vi "Enable-disable control.vi"(8 "error in":errorcluster, 10 "Status":T1(array[ring]), 11 "Ref array":refnum<vi>[](array[refnum])) -> (0 "error out":errorcluster)   [LabVIEW 2018]
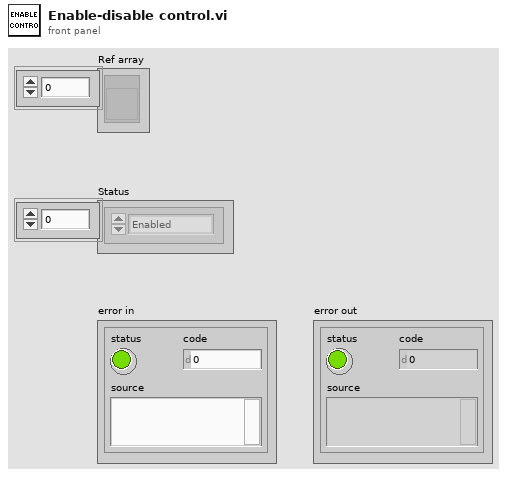
[diagram p1: front panel]
types:
  T1 = enum8{"Enabled", "Disabled", "Disabled and Grayed Out"}[]
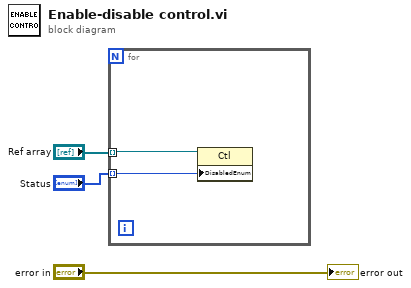
[diagram p0: block diagram]
diagram:
  n1 = for {
    tunnel: "Ref array" -> [w5] mode=indexing
    tunnel: "Status" -> [w4] mode=indexing
    n2 = property class="Ctl"(reference=w5, "DisabledEnum"=w4) -> ()  [unwired: 1 in, 2 out]
  }
  "error out" <- "error in"
